vi "Geometry prep.vi"() -> ()   [LabVIEW 2015]
uses:
  <vilib>/Analysis/NI_AALPro.lvlib
panel:
  out "Area vectors, cylinder (sorted)":sgl[][](array[numeric])=[[-0.0029639693, -0.0012277163, -0.0], [-0.002545218, -0.0019530145, -0.0], [-0.0019530145, -0.002545218, -0.0], [-0.0012277163, -0.0029639693, -0.0], [-0.0, -0.0063614617, -0.0], [0.0012277163, -0.0029639693, 0.0], [0.0019530145, -0.002545218, 0.0], [0.002545218, -0.0019530145, 0.0], [0.0029639693, -0.0012277163, 0.0], [0.0063614617, 0.0, 0.0], [0.0029639693, 0.0012277163, 0.0], [0.002545218, 0.0019530145, 0.0], [0.0019530145, 0.002545218, 0.0], [0.0012277163, 0.0029639693, 0.0], [-0.0, 0.0063614617, 0.0], [-0.0012277163, 0.0029639693, 0.0], [-0.0019530145, 0.002545218, 0.0], [-0.002545218, 0.0019530145, 0.0], [-0.0029639693, 0.0012277163, 0.0], [-0.0063614617, 0.0, 0.0]]
  in  "Span (m)":dbl=0.43
  in  "Radius (m)":dbl=0.02858
  in  "Clockwise winding?":bool
  in  "y/c cylinder (sorted":dbl[](array[numeric])=[0.258819043636322, 0.5, 0.7071067690849304, 0.8660253882408142, 0.9659258127212524, 0.9659258127212524, 0.8660253882408142, 0.7071067690849304, 0.5, 0.258819043636322, -0.258819043636322, -0.5, -0.7071067690849304, -0.8660253882408142, -0.9659258127212524, -0.9659258127212524, -0.8660253882408142, -0.7071067690849304, -0.5, -0.258819043636322]
  in  "x/c cylinder (sorted)":dbl[](array[numeric])=[0.9659258127212524, 0.8660253882408142, 0.7071067690849304, 0.5, 0.258819043636322, -0.258819043636322, -0.5, -0.7071067690849304, -0.8660253882408142, -0.9659258127212524, -0.9659258127212524, -0.8660253882408142, -0.7071067690849304, -0.5, -0.258819043636322, 0.258819043636322, 0.5, 0.7071067690849304, 0.8660253882408142, 0.9659258127212524]
  # "(Data sorted by winding no.)"
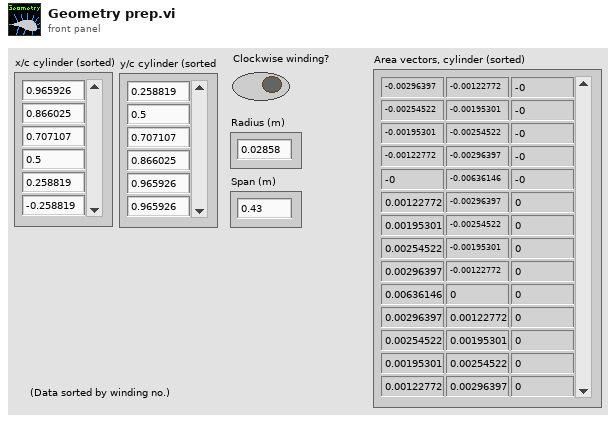
[diagram p1: front panel]
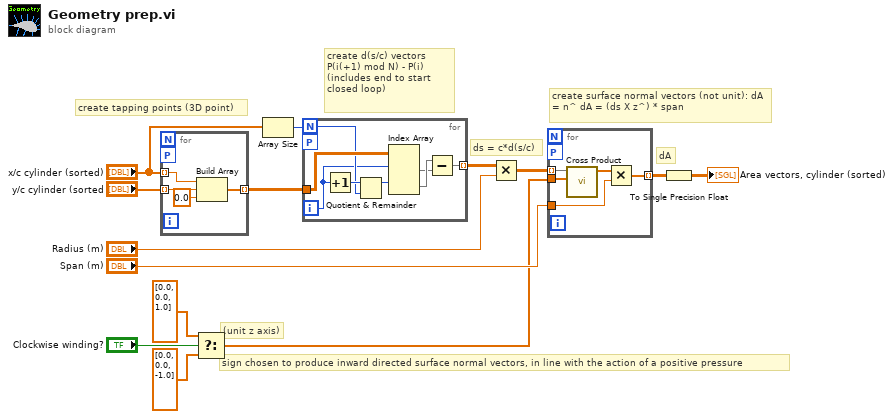
[diagram p0: block diagram]
diagram:
  # "sign chosen to produce inward directed surface normal vectors, in line with the action of a positive pressure"
  # "(unit z axis)"
  # "dA"
  # "create surface normal vectors (not unit): dA = n^ dA = (ds X z^) * span"
  # "ds = c*d(s/c)"
  # "create d(s/c) vectors P(i(+1) mod N) - P(i)\n(includes end to start closed loop)"
  # "create tapping points (3D point)"
  n1 = for {
    workers-P: _ -> [_]
    tunnel: "x/c cylinder (sorted)" -> [w18] mode=indexing
    tunnel: "y/c cylinder (sorted" -> [w17] mode=indexing
    tunnel: [w15] -> w9 mode=indexing
    n2 = Build Array(w18, w17, 0.0 ("element")) -> (w15:dbl[])
  }
  n3 = Select(t=dbl[] [0.0, 0.0, 1.0], s="Clockwise winding?", f=dbl[] [0.0, 0.0, -1.0]) -> (s? t:f=w2:dbl[])
  n4 = Array Size(array="x/c cylinder (sorted)") -> (size(s)=w1:i32)
  n5 = for {
    N: w1 -> [w20]
    tunnel: w9 -> [w25]
    tunnel: [w26] -> w8 mode=indexing
    workers-P: _ -> [_]
    i -> [w19]
    n6 = Increment(x=w19) -> (x+1=w21:i32)
    n7 = Quotient & Remainder(x=w21, y=w20) -> (x-y*floor(x/y)=w22:i32)  [unwired: 1 out]
    n8 = Index Array(array=w25, index (row) #1=w19, index (row) #2=w22) -> (element #1=w23:dbl[], element #2=w24:dbl[])  [unwired: 2 in]
    n9 = Subtract(x=w24, y=w23) -> (x-y=w26:dbl[])
  }
  n10 = Multiply(x=w8, y="Radius (m)") -> (x*y=w6:dbl[][])
  n11 = for {
    tunnel: w6 -> [w31] mode=indexing
    tunnel: w2 -> [w30]
    workers-P: _ -> [_]
    tunnel: "Span (m)" -> [w28]
    tunnel: [w27] -> w4 mode=indexing
    n12 = call <vilib>:"Cross Product.vi"("B Vector"=w30, "A Vector"=w31) -> ("Cross Product"=w29:dbl[])  [unwired: 8 in, 1 out]
    n13 = Multiply(x=w29, y=w28) -> (x*y=w27:dbl[])
  }
  n14 = To Single Precision Float(number=w4) -> (single precision float=→"Area vectors, cylinder (sorted)":sgl[][])
